vi "Read Holding Registers.vi"(8 "error in (no error)":errorcluster, 9 "number of registers":u16, 10 "starting address":u16, 11 "standard data model in":refnum<class "ICPCON ET Data Model.lvclass">) -> (0 "error out":errorcluster, 2 "data":u16[](array[numeric]), 3 "standard sata model out":refnum<class "ICPCON ET Data Model.lvclass">)   [LabVIEW 2021, in "ICPCON ET Data Model.lvclass"]
doc: "Reads N holding registers from the device model, starting at register M."
uses:
  ICPCON ET Data Model.lvclass
  ICPCON ET Data Model.lvclass/ICPCON ET Data Model.ctl
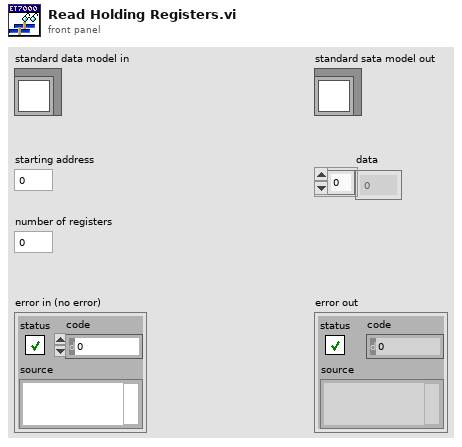
[diagram p1: front panel]
types:
  T1 = typedef "ICPCON ET Data Model.lvclass/Data Model.ctl" = cluster{"UTC":u64, "DI":bool[], "DO":bool[], "IR":u16[], "HR":u16[], "ES":u8}
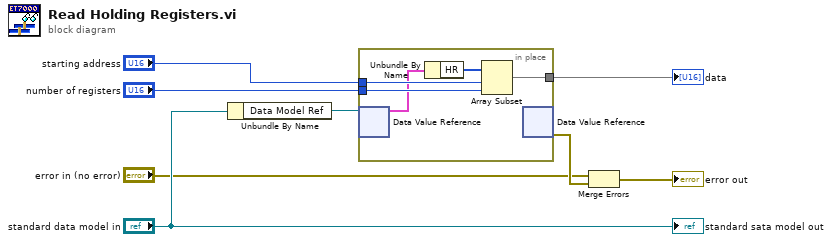
[diagram p0: block diagram]
diagram:
  n1 = Unbundle By Name("standard data model in") -> ("Data Model Ref"=w3:refnum<data-value>)
  n2 = in-place {
    in-place-border: [w13] -> w6
    in-place-border: "starting address" -> [w12]
    in-place-border: "number of registers" -> [w11]
    n3 = in-place-dvr #1(w3) -> (w10:T1)  [unwired: 1 out]
    n4 = Unbundle By Name(w10) -> ("HR"=w9:u16[])
    n5 = Array Subset(array=w9, index=w12, length=w11) -> (w13:u16[])
    n6 = in-place-dvr #1() -> (w2:errorcluster)  [unwired: 1 in, 1 out]
  }
  "data" <- w6
  n7 = Merge Errors("error in (no error)", w2) -> (→"error out":errorcluster)
  "standard sata model out" <- "standard data model in"
